vi "MGI RWA Write Strings to File.vi"(8 "Error In":errorcluster, 9 "Section Name":string, 10 "Strings[]":string[](array[string]), 11 "Path":path) -> (0 "Error Out":errorcluster, 2 "Section Replaced?":bool)   [LabVIEW 2020]
doc: "This VI was created for use with the Read/Write Cluster VIs. It writes the cluster element strings to the specified section in an INI file without editing any other sections.\n\nAuthored by Robert C. Mortensen\nsupport@mooregoodideas.com\nwww.mooregoodideas.com\n\nCopyright (c) 2010, Moore Good Ideas, Inc.\n\nAll rights reserved.\n\nRedistribution and use in source and binary forms, with or without modification, are permitted provided that the following conditions are met:\n\n * Redistributions of source code must retain the above copyright notice, this list of conditions and the following disclaimer.\n * Redistributions in binary form must reproduce the above copyright notice, this list of conditions and the following disclaimer in the documentation and/or other materials provided with the distribution.\n * Neither the name of Moore Good Ideas, Inc. nor the names of its contributors may be used to endorse or promote products derived from this software without specific prior written permission.\n\nTHIS SOFTWARE IS PROVIDED BY THE COPYRIGHT HOLDERS AND CONTRIBUTORS \"AS IS\" AND ANY EXPRESS OR IMPLIED WARRANTIES, INCLUDING, BUT NOT LIMITED TO, THE IMPLIED WARRANTIES OF MERCHANTABILITY AND FITNESS FOR A PARTICULAR PURPOSE ARE DISCLAIMED. IN NO EVENT SHALL THE COPYRIGHT OWNER OR CONTRIBUTORS BE LIABLE FOR ANY DIRECT, INDIRECT, INCIDENTAL, SPECIAL, EXEMPLARY, OR CONSEQUENTIAL DAMAGES (INCLUDING, BUT NOT LIMITED TO, PROCUREMENT OF SUBSTITUTE GOODS OR SERVICES; LOSS OF USE, DATA, OR PROFITS; OR BUSINESS INTERRUPTION) HOWEVER CAUSED AND ON ANY THEORY OF LIABILITY, WHETHER IN CONTRACT, STRICT LIABILITY, OR TORT (INCLUDING NEGLIGENCE OR OTHERWISE) ARISING IN ANY WAY OUT OF THE USE OF THIS SOFTWARE, EVEN IF ADVISED OF THE POSSIBILITY OF SUCH DAMAGE."
uses:
  <userlib>/_MGI/Error Handling/MGI Suppress Error Code/MGI Suppress Error Code (Scalar).vi
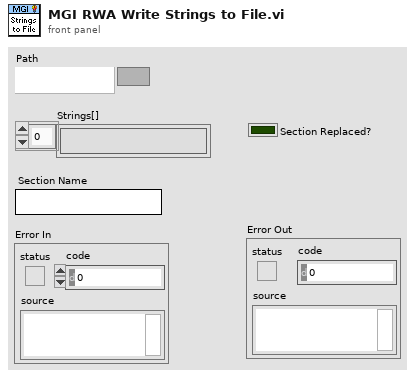
[diagram p1: front panel]
types:
  T1 = enum16{"Auto Detect", "Path Contains a File", "Path Does Not Contain a File"}
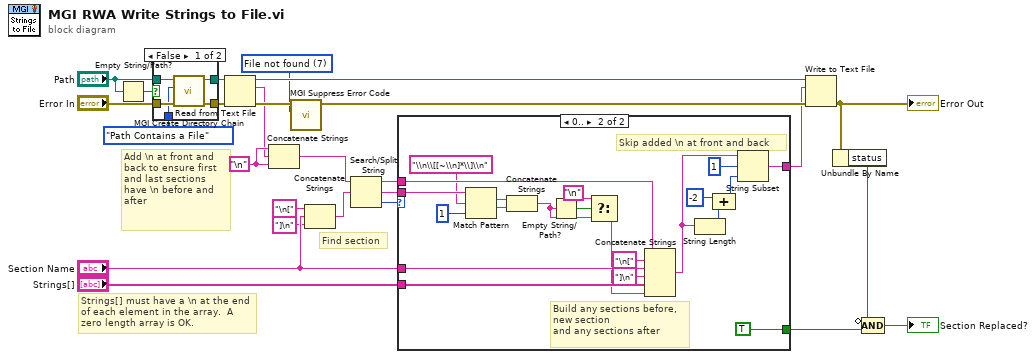
[diagram p0: block diagram]
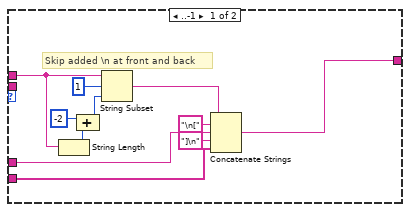
[diagram p2: hidden frame]
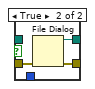
[diagram p3: hidden frame]
diagram:
  w10 = u16 7 items=["No error", "Argument error", "Memory is full", "Out of zone", "End of file", "File already open", "Generic file I/O error", "File not found", "File permission error", "Disk is full", "Duplicate path", "Too many files open", "System feature not enabled", "Resource file not found", "Cannot add resource", "Resource not found", "Image not found", "Image memory error", "Pen does not exist", "Config type invalid", "Config token not found", "Config parse error", "Config memory error", "Bad external code format", "Bad external code offset", "External code not present", "Null window", "Destroy window error", "Null menu", "Print aborted", "Bad print record", "Print driver error", "Windows error during printing", "Memory error during printing", "Print dialog error", "Generic print error", "Invalid device refnum", "Device not found", "Device parameter error", "Device unit error", "Cannot open device", "Device call aborted", "Generic error", "Cancelled by user", "Object ID too low", "Object ID too high", "Object not in heap", "Unknown heap", "Unknown object (invalid DefProc)", "Unknown object (DefProc not in table)", "Message out of range", "Invalid (null) method", "Unknown message", "Manager call not supported", "Bad address", "Network operation in progress", "Network operation timed out", "Connection is busy", "Network attribute not supported", "Network error", "Address in use", "System out of memory", "Connection aborted", "Connection refused", "Not connected", "Already connected", "Connection closed", "Initialization error (interapplication manager)", "Bad occurrence", "Wait on unbound occurrence handler", "Occurrence queue overflow", "Datalog type conflict", "Unused", "Unrecognized type (interapplication manager)", "Memory corrupt", "Failed to make temporary DLL", "Old CIN version", "Drag socket not found", "Failed to load drop-object", "Failed to register OLE object", "Failed to release OLE object", "Format specifier type mismatch", "Unknown format specifier", "Too few format specifiers", "Too many format specifiers", "Scan failed", "Newer CIN version", "OLE Convert", "Runtime menu error", "Password tampered", "Unknown error code"] ("Reserved Error Code (Generic error)")
  w16 = "\n"
  # "Add \\n at front and back to ensure first and last sections have \\n before and after"
  # "Strings[] must have a \\n at the end of each element in the array.  A zero length array is OK."
  # "Find section"
  n1 = Empty String/Path?(string/path="Path") -> (empty?=w17:bool)
  n2 = case shown="False" w17 {
    tunnel: "Error In" -> [w30 w33]
    tunnel: [w29 w32] -> w20
    tunnel: [w28 w31] -> w19
    tunnel: "Path" -> [w27 _]
    tunnel: T1."Path Contains a File" ("File Presence (Auto Detect)") -> [w26 _]
    frame False {
      n3 = call <userlib>:"MGI Create Directory Chain.vi"("Error In"=w30, "File Presence (Auto Detect)"=w26, "Path"=w27) -> ("Error Out"=w29:errorcluster, "Duplicate Path"=w28:path)  [unwired: 7 out]
    }
    frame True {
      n4 = File Dialog(8:w33) -> (0:w32:errorcluster, 3:w31:path)  [unwired: 8 out]
    }
  }
  n5 = Read from Text File(file (use dialog)=w19, error in=w20) -> (text=w6:string, error out=w14:errorcluster)  [unwired: 4 out]
  n6 = Concatenate Strings(w16, w6, w16) -> (w12:string)
  n7 = call-poly <userlib>:"MGI Suppress Error Code.vi"("Error Code"=w10, "Error In"=w14) -> ("Error Out"=w13:errorcluster)  [unwired: 4 in, 1 out]
  n8 = Concatenate Strings("\n[" ("string"), "Section Name", "]\n" ("string")) -> (w11:string)
  n9 = Search/Split String(string=w12, search string/char (-)=w11) -> (substring before match=w9:string, match + rest of string=w7:string, offset of match=w5:i32)  [unwired: 1 in]
  n10 = case shown="0.." w5 {
    tunnel: "Section Name" -> [w42 w65]
    tunnel: "Strings[]" -> [w41 w64]
    tunnel: w9 -> [w35 w63]
    tunnel: [w40 w61] -> w8
    tunnel: w7 -> [_ w56]
    tunnel: [_ TRUE] -> w2
    frame ..-1 {
      # "Skip added \\n at front and back"
      n11 = String Length(string=w35) -> (length=w38:i32)
      n12 = Compound Arithmetic op=ADD(-2 ("value"), w38) -> (w37:i32)
      n13 = String Subset(string=w35, offset (0)=1, length (rest)=w37) -> (substring=w34:string)
      n14 = Concatenate Strings(w34, "\n[" ("string"), w42, "]\n" ("string"), w41) -> (w40:string)
    }
    frame 0.. {
      # "Build any sections before,\nnew section\nand any sections after"
      # "Skip added \\n at front and back"
      n15 = Match Pattern(string=w56, regular expression="\\n\\[[~\\n]*\\]\\n", offset (0)=1) -> (match substring=w50:string, after substring=w49:string)  [unwired: 2 out]
      n16 = Concatenate Strings(w50, w49) -> (w47:string)
      n17 = Empty String/Path?(string/path=w47) -> (empty?=w52:bool)
      n18 = Select(t="\n", s=w52, f=w47) -> (s? t:f=w51:string)
      n19 = Concatenate Strings(w63, "\n[" ("string"), w65, "]\n" ("string"), w64, w51) -> (w62:string)
      n20 = String Length(string=w62) -> (length=w59:i32)
      n21 = Compound Arithmetic op=ADD(-2 ("value"), w59) -> (w58:i32)
      n22 = String Subset(string=w62, offset (0)=1, length (rest)=w58) -> (substring=w61:string)
    }
  }
  n23 = Write to Text File(file (use dialog)=w19, text=w8, error in=w13) -> (error out=w4:errorcluster)  [unwired: 3 out]
  "Error Out" <- w4
  n24 = Unbundle By Name(w4) -> ("status"=w3:bool)
  n25 = Compound Arithmetic op=AND(invert w3, w2) -> (→"Section Replaced?":bool)
